vi "SAL Connect User Dialog.vi"(8 "error in (no error)":errorcluster, 9 "M1M3 Support Events in":refnum<class "M1M3 Support Events.lvclass">, 11 "SAL in":refnum<class "SAL.lvclass">) -> (0 "error out":errorcluster, 3 "SAL out":refnum<class "SAL.lvclass">)   [LabVIEW 2016, in "SAL.lvclass"]
uses:
  SAL.lvclass
  M1M3 Support Events/M1M3 Support Events.lvclass
  M1M3 Support Events/M1M3 Support Events.lvclass/M1M3 Support Events.ctl
panel:
  # "Connecting to SAL.   Please Wait...."
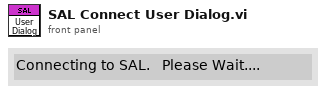
[diagram p1: front panel]
types:
  T1 = typedef "M1M3SupportEUI_TypeDefs.lvlib/M1M3 Support Events.ctl" = cluster{"M1M3 Support State":refnum<user-event>, "Inclinometer  Data":refnum<user-event>, "IMS Data":refnum<user-event>, "FA Data":refnum<user-event>, "FA Status":refnum<user-event>, "SAL Connected":refnum<user-event>, "HP Data":refnum<user-event>, "HP Status":refnum<user-event>}
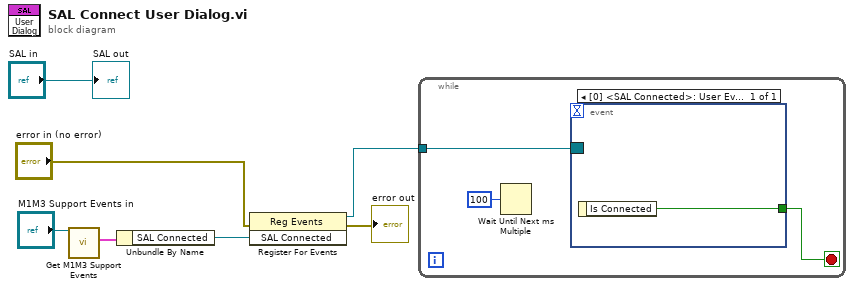
[diagram p0: block diagram]
diagram:
  n1 = call "Get M1M3 Support Events.vi"("M1M3 Support Events in"="M1M3 Support Events in") -> ("M1M3 Support Events"=w5:T1)  [unwired: 9 in, 1 out]
  n2 = Unbundle By Name(w5) -> ("SAL Connected"=w4:refnum<user-event>)
  n3 = register-events(error in="error in (no error)", w4) -> (reference out=w3:refnum<event-registration>, error out=→"error out":errorcluster)  [unwired: 1 in]
  n4 = while {
    tunnel: w3 -> [w10]
    stop <- w9 stop-if-true
    n5 = Wait Until Next ms Multiple(millisecond multiple=u32 100) -> ()  [unwired: 1 out]
    n6 = event shown="[0] <SAL Connected>: User Event" {
      selector: w10 -> [_]
      dyn-events: _ -> [_]
      timeout: _ -> [_]
      tunnel: [w11] -> w9
      event User Event {
        n7 = event-data() -> ("Is Connected"=w11:bool)  [unwired: 1 in]
      }
    }
  }
  "SAL out" <- "SAL in"
